vi "heating_ZM_state_ind.vi"(10 "Z_State":T1=enum."on", 11 "Z_Source":T2=enum."local disabled") -> (3 "N ring":u16)   [LabVIEW 2019, in "Heating.lvlib"]
uses:
  Heating.lvlib
  ctl/Z_source.ctl
  ctl/Z_State.ctl
  Counter/Counter.lvlib
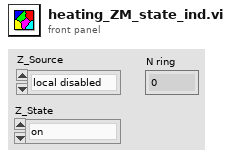
[diagram p1: front panel]
types:
  T1 = typedef "Heating.lvlib/Z_State.ctl" = enum8{"initialization", "alarm", "disabled", "not ready", "stop ready", "reserv", "switched off", "reserv2", "switched on", "check", "on min", "decrease out", "on", "increase out", "on max"}
  T2 = typedef "Heating.lvlib/Z_source.ctl" = enum8{"initialize", "local disabled", "local hand", "hand", "auto", "dist"}
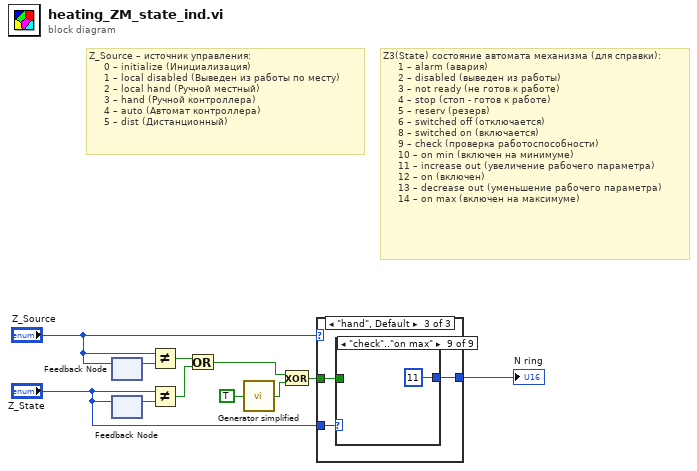
[diagram p0: block diagram]
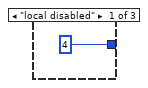
[diagram p2: hidden frame]
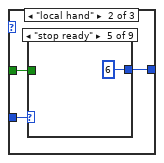
[diagram p3: hidden frame]
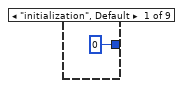
[diagram p4: hidden frame]
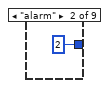
[diagram p5: hidden frame]
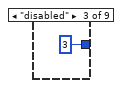
[diagram p6: hidden frame]
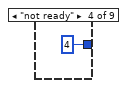
[diagram p7: hidden frame]
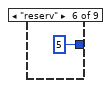
[diagram p8: hidden frame]
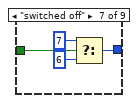
[diagram p9: hidden frame]
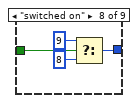
[diagram p10: hidden frame]
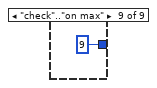
[diagram p11: hidden frame]
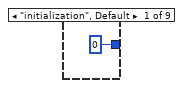
[diagram p12: hidden frame]
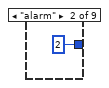
[diagram p13: hidden frame]
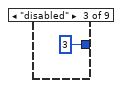
[diagram p14: hidden frame]
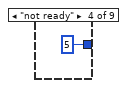
[diagram p15: hidden frame]
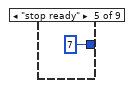
[diagram p16: hidden frame]
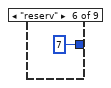
[diagram p17: hidden frame]
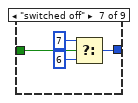
[diagram p18: hidden frame]
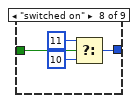
[diagram p19: hidden frame]
diagram:
  # "Z_Source – источник управления:\n     0 – initialize (Инициализация)\n     1 – local disabled (Выведен из работы по месту)\n     2 – local hand (Ручной местный)\n     3 – hand (Ручной контроллера)\n     4 – auto (Автомат контроллера)\n     5 – dist (Дистанционный)"
  # "Z3(State) состояние автомата механизма (для справки):\n     1 – alarm (авария)\n     2 – disabled (выведен из работы)\n     3 – not ready (не готов к работе)\n     4 – stop (стоп - готов к работе)\n     5 – reserv (резерв)\n     6 – switched off (отключается)\n     8 – switched on (включается)\n     9 – check (проверка работоспособности)\n     10 – on min (включен на минимуме)\n     11 – increase out (увеличение рабочего параметра)\n     12 – on (включен)\n     13 – decrease out (уменьшение рабочего параметра)\n     14 – on max (включен на максимуме)"
  n1 = feedback #1() -> (w11:T2)  [unwired: 1 in]
  n2 = feedback-in #1("Z_Source") -> ()
  n3 = feedback #2() -> (w10:T1)  [unwired: 1 in]
  n4 = feedback-in #2("Z_State") -> ()
  n5 = Not Equal?(x="Z_Source", y=w11) -> (x != y?=w9:bool)
  n6 = Not Equal?(x="Z_State", y=w10) -> (x != y?=w8:bool)
  n7 = Or(x=w9, y=w8) -> (x .or. y?=w2:bool)
  n8 = call "Generator simplified.vi"("ON (F)"=TRUE) -> ("Q"=w4:bool)
  n9 = Exclusive Or(1:w4, 2:w2) -> (0:w3:bool)
  n10 = case shown="\"hand\", Default" "Z_Source" {
    tunnel: w3 -> [_ w15 w32]
    tunnel: "Z_State" -> [_ w14 w33]
    tunnel: [u16 4 ("Z5 ind") w13 w31] -> w1
    frame "local disabled" {
    }
    frame "local hand" {
      n11 = case shown="\"stop ready\"" w14 {
        tunnel: [u16 0 ("Z5 ind") u16 2 ("Z5 ind") u16 3 ("Z5 ind") u16 4 ("Z5 ind") u16 6 ("Z5 ind") u16 5 ("Z5 ind") w23 w27 u16 9 ("Z5 ind")] -> w13
        tunnel: w15 -> [_ _ _ _ _ _ w22 w26 _]
        frame "initialization", Default {
        }
        frame "alarm" {
        }
        frame "disabled" {
        }
        frame "not ready" {
        }
        frame "stop ready" {
        }
        frame "reserv" {
        }
        frame "switched off" {
          n12 = Select(t=u16 7 ("Z5 ind"), s=w22, f=u16 6) -> (s? t:f=w23:u16)
        }
        frame "switched on" {
          n13 = Select(t=u16 9 ("Z5 ind"), s=w26, f=u16 8) -> (s? t:f=w27:u16)
        }
        frame "check".."on max" {
        }
      }
    }
    frame "hand", Default {
      n14 = case shown="\"check\"..\"on max\"" w33 {
        tunnel: [u16 0 ("Z5 ind") u16 2 ("Z5 ind") u16 3 ("Z5 ind") u16 5 ("Z5 ind") u16 7 ("Z5 ind") u16 7 ("Z5 ind") w41 w45 u16 11 ("Z5 ind")] -> w31
        tunnel: w32 -> [_ _ _ _ _ _ w40 w44 _]
        frame "initialization", Default {
        }
        frame "alarm" {
        }
        frame "disabled" {
        }
        frame "not ready" {
        }
        frame "stop ready" {
        }
        frame "reserv" {
        }
        frame "switched off" {
          n15 = Select(t=u16 7 ("Z5 ind"), s=w40, f=u16 6) -> (s? t:f=w41:u16)
        }
        frame "switched on" {
          n16 = Select(t=u16 11 ("Z5 ind"), s=w44, f=u16 10) -> (s? t:f=w45:u16)
        }
        frame "check".."on max" {
        }
      }
    }
  }
  "N ring" <- w1
